vi "Compute Line Rate.vi"(8 "error in (no error)":errorcluster, 11 "Package in":refnum<class "Package.lvclass">) -> (0 "error out":errorcluster, 3 "Package out":refnum<class "Package.lvclass">)   [LabVIEW 2017, in "Cobertura.lvlib" / "Package.lvclass"]
uses:
  Package.lvclass
  Package.lvclass/Package.ctl
  Class/Class.lvclass/Class.ctl
  Class/Read Line Rate.vi
  Class/Class.lvclass
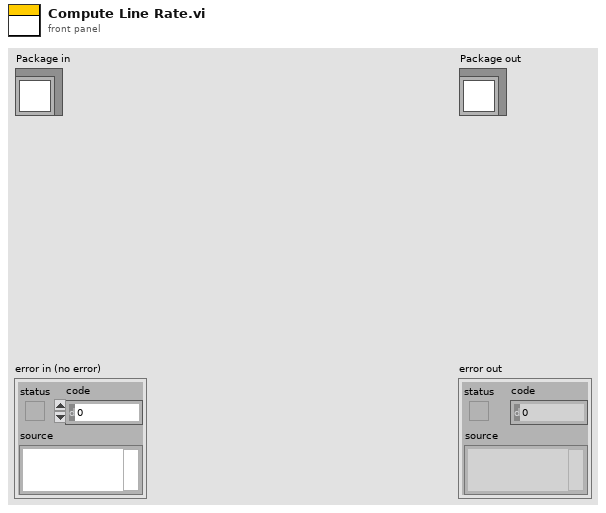
[diagram p1: front panel]
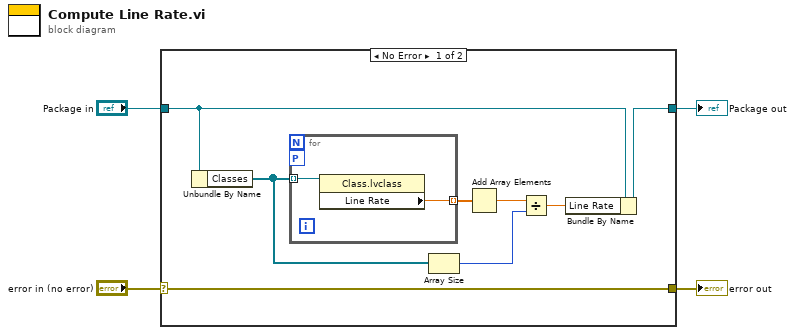
[diagram p0: block diagram]
diagram:
  n1 = case shown="No Error" "error in (no error)" {
    selector: "error in (no error)" -> [w12 w16]
    tunnel: [w12 w16] -> w3
    tunnel: [w5 w15] -> w1
    tunnel: "Package in" -> [w6 w15]
    frame No Error {
      n2 = Unbundle By Name(w6) -> ("Classes"=w9:refnum<class "Class.lvclass">[])
      n3 = for {
        tunnel: w9 -> [w14] mode=indexing
        tunnel: [w13] -> w11 mode=indexing
        workers-P: _ -> [_]
        n4 = property class="Class.lvclass"(reference=w14) -> ("Line Rate"=w13:dbl)  [unwired: 1 in, 2 out]
      }
      n5 = Array Size(array=w9) -> (size(s)=w8:i32)
      n6 = Add Array Elements(numeric array=w11) -> (sum=w10:dbl)
      n7 = Divide(x=w10, y=w8) -> (x/y=w7:dbl)
      n8 = Bundle By Name(cluster=w6, "Line Rate"=w7) -> (w5:refnum<class "Package.lvclass">)
    }
    frame Error {
    }
  }
  "error out" <- w3
  "Package out" <- w1
